vi "Connected.vi"(8 "error in (no error)":errorcluster, 11 "GodotServer in":refnum<class "GodotServer.lvclass">) -> (0 "error out":errorcluster, 2 "Connected":bool, 3 "GodotServer out":refnum<class "GodotServer.lvclass">)   [LabVIEW 2020, in "GodotLV.lvlib" / "GodotServer.lvclass"]
doc: "Returns True when a client has connected to the WebSocket stream."
uses:
  GodotServer.lvclass
  GodotServer.lvclass/GodotServer.ctl
  <vilib>/IlluminatedG/IG WebSocket Stream/Stream-Websocket/Websocket Server/Websocket Server.lvclass
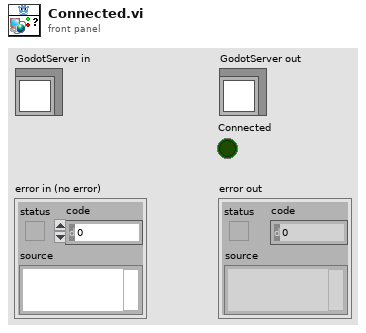
[diagram p1: front panel]
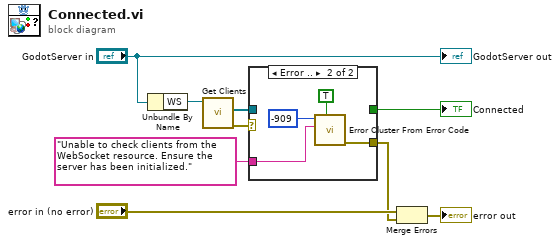
[diagram p0: block diagram]
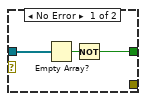
[diagram p2: hidden frame]
diagram:
  n1 = Unbundle By Name("GodotServer in") -> ("WS"=w7:refnum<class "Websocket Server.lvclass">)
  n2 = call <vilib>:"Get Clients.vi"("Websocket Server in"=w7) -> ("error out"=w5:errorcluster, "Clients"=w6:refnum<class "Websocket Client.lvclass">[])  [unwired: 8 in, 1 out]
  n3 = case shown="Error .." w5 {
    tunnel: w6 -> [w12 _]
    tunnel: [w10 _] -> w4
    tunnel: "Unable to check clients from the WebSocket resource. Ensure the server has been initialized." ("error message (\"\")") -> [_ w14]
    tunnel: [_ w13] -> w1
    frame No Error {
      n4 = Empty Array?(array=w12) -> (empty?=w11:bool)
      n5 = Not(x=w11) -> (.not. x?=w10:bool)
    }
    frame Error {
      n6 = call <vilib>:"Error Cluster From Error Code.vi"("show call chain? (False)"=TRUE, "error message (\"\")"=w14, "error code (0)"=-909) -> ("error out"=w13:errorcluster)  [unwired: 6 in]
    }
  }
  "Connected" <- w4
  n7 = Merge Errors("error in (no error)", w1) -> (→"error out":errorcluster)
  "GodotServer out" <- "GodotServer in"
